vi "Variant Checksum.vi"(2 "Variant":variant) -> (7 "Checksum":u64)   [LabVIEW 2021, in "Variant.lvlib"]
uses:
  Variant.lvlib
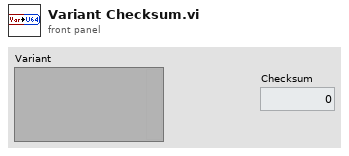
[diagram p1: front panel]
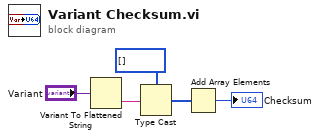
[diagram p0: block diagram]
diagram:
  n1 = Variant To Flattened String(Variant="Variant") -> (data string=w3:string)  [unwired: 1 out]
  n2 = Type Cast(type=u64[] [] ("Bin"), x=w3) -> (*(type *) &x=w5:u64[])
  n3 = Add Array Elements(numeric array=w5) -> (sum=→"Checksum":u64)
